vi "TurnON_OFF_DAC_1212.vi"(2 "error in (no error)":errorcluster, 3 "TurnON":bool, 4 "Selected DAC":u8(ring) items=["DAC0 (A)", "DAC1 (B)"], 5 "FPGA Interface In":refnum<k20>) -> (0 "error out":errorcluster, 1 "FPGA Interface Out":refnum<k20>)   [LabVIEW 2018]
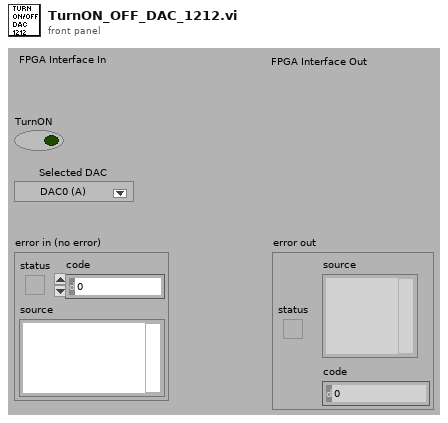
[diagram p1: front panel]
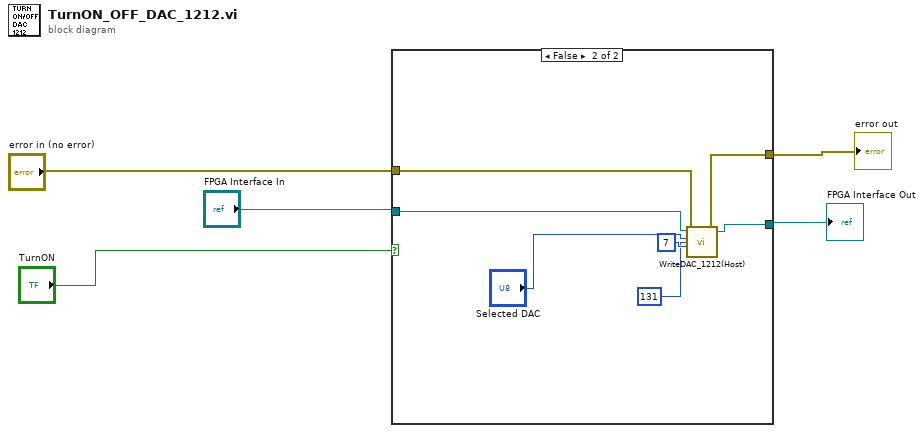
[diagram p0: block diagram]
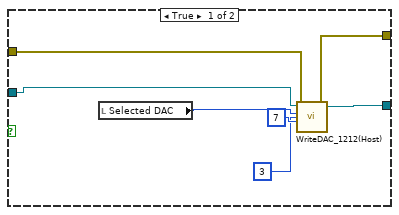
[diagram p2: hidden frame]
diagram:
  n1 = case shown="False" "TurnON" {
    tunnel: [w10 w17] -> w1
    tunnel: "error in (no error)" -> [w8 w15]
    tunnel: [w9 w16] -> w4
    tunnel: "FPGA Interface In" -> [w7 w14]
    frame True {
      n2 = local read "Selected DAC"() -> (w6:u8)
      n3 = call "WriteDAC_1212(Host).vi"("FPGA Interface In"=w7, "Selected DAC"=w6, "Address"=u8 7 ("Adress"), "error in (no error)"=w8, "Data"=u8 3) -> ("FPGA Interface Out"=w10:refnum<k20>, "error out"=w9:errorcluster)  [unwired: 1 in]
    }
    frame False {
      n4 = call "WriteDAC_1212(Host).vi"("FPGA Interface In"=w14, "Selected DAC"="Selected DAC", "Address"=u8 7 ("Adress"), "error in (no error)"=w15, "Data"=u8 131) -> ("FPGA Interface Out"=w17:refnum<k20>, "error out"=w16:errorcluster)  [unwired: 1 in]
    }
  }
  "error out" <- w4
  "FPGA Interface Out" <- w1
